vi "Split Log.vi"(8 "error in (no error)":errorcluster, 11 "Event Reporter Module in":refnum<class "Event Reporter Module.lvclass">) -> (0 "error out":errorcluster, 3 "Event Reporter Module out":refnum<class "Event Reporter Module.lvclass">)   [LabVIEW 2020, in "Volatus.lvlib" / "Event Reporter Module.lvclass"]
uses:
  Event Reporter Module.lvclass
  Event Reporter Module.lvclass/Event Reporter Module.ctl
  Event Level.ctl
  Volatus.lvlib
  Event.ctl
  Module/Module.lvclass
  C:/dev/lv20CE/relink/lv-volatus/Volatus/Module/Module.lvclass
  C:/dev/lv20CE/relink/lv-volatus/Volatus/Event Reporter Module/Event Reporter Module.lvclass
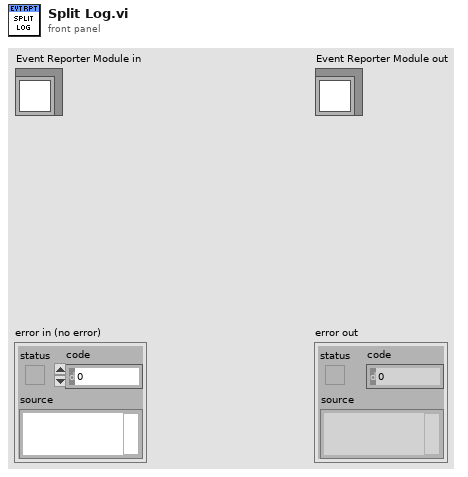
[diagram p1: front panel]
types:
  T1 = typedef "Volatus.lvlib/Event Level.ctl" = enum16{"Debug", "Info", "Warning", "Error"}
  T2 = typedef "Volatus.lvlib/Event.ctl" = cluster{"Time Stamp":timestamp, "Event Level":T1, "Context":string, "Message":string, "Error":errorcluster}
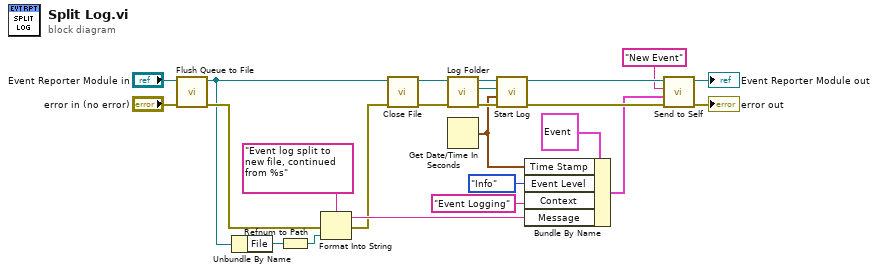
[diagram p0: block diagram]
diagram:
  n1 = call "Flush Queue to File.vi"("error in (no error)"="error in (no error)", "Event Reporter Module in"="Event Reporter Module in") -> ("error out"=w24:errorcluster, "Event Reporter Module out"=w6:refnum<class "Event Reporter Module.lvclass">)  [unwired: 8 in]
  n2 = Unbundle By Name(w6) -> ("File"=w5:refnum<file>)
  n3 = Refnum to Path(1:w5) -> (0:w4:path)
  n4 = Format Into String(format string="Event log split to new file, continued from %s" ("Message"), error in=w24, w4) -> (resulting string=w3:string, error out=w2:errorcluster)  [unwired: 1 in]
  n5 = call "Close File.vi"("error in (no error)"=w2, "Event Reporter Module in"=w6) -> ("error out"=w22:errorcluster, "Event Reporter Module out"=w19:refnum<class "Event Reporter Module.lvclass">)  [unwired: 8 in]
  n6 = call "Log Folder.vi"("error in (no error)"=w22, "Event Reporter Module in"=w19) -> ("error out"=w20:errorcluster, "Log Folder"=w17:path, "Event Reporter Module out"=w18:refnum<class "Event Reporter Module.lvclass">)  [unwired: 7 in]
  n7 = Get Date/Time In Seconds() -> (seconds since 1Jan1904=w9:timestamp)
  n8 = call "Start Log.vi"("error in (no error)"=w20, "Time Stamp"=w9, "Folder"=w17, "Event Reporter Module in"=w18) -> ("error out"=w21:errorcluster, "Event Reporter Module out"=w15:refnum<class "Event Reporter Module.lvclass">)  [unwired: 6 in]
  n9 = Bundle By Name(cluster=T2 {"Time Stamp"=timestamp(0 s since 1904-01-01), "Event Level"=enum."Info", "Context"="", "Message"="", "Error"={"status"=FALSE, "code"=0, "source"=""}} ("Event"), "Time Stamp"=w9, "Event Level"=Event_Level."Info", "Context"="Event Logging", "Message"=w3) -> (w8:T2)
  n10 = call "Send to Self.vi"("error in (no error)"=w21, "Data"=w8, "Message ID"="New Event", "Module in"=w15) -> ("error out"=→"error out":errorcluster, "Module out"=→"Event Reporter Module out":refnum<class "Event Reporter Module.lvclass">)  [unwired: 6 in]
